vi "stageTriggerCam.vi"() -> ()   [LabVIEW 2015]
panel:
  in  "initTrigPos (mm)":dbl
  out "Frame Count":i32=1
  in  "File":path=path "C:/Users/sims01/Desktop/triggering1711/imgStack"
  in  "System no.":i32=2 min=1 step=1
  in  "zIdx":i32=1
  in  "error in":errorcluster
  in  "triggOutputIdx":string="3"
  in  "initPos (mm)":dbl
  in  "finPos (mm)":dbl=10.0
  in  "stepSize (mm)":dbl=0.5
  in  "motionSelection":enum32{"stop/ start", "cont."}(radio)=enum."cont."
  out "error out":errorcluster
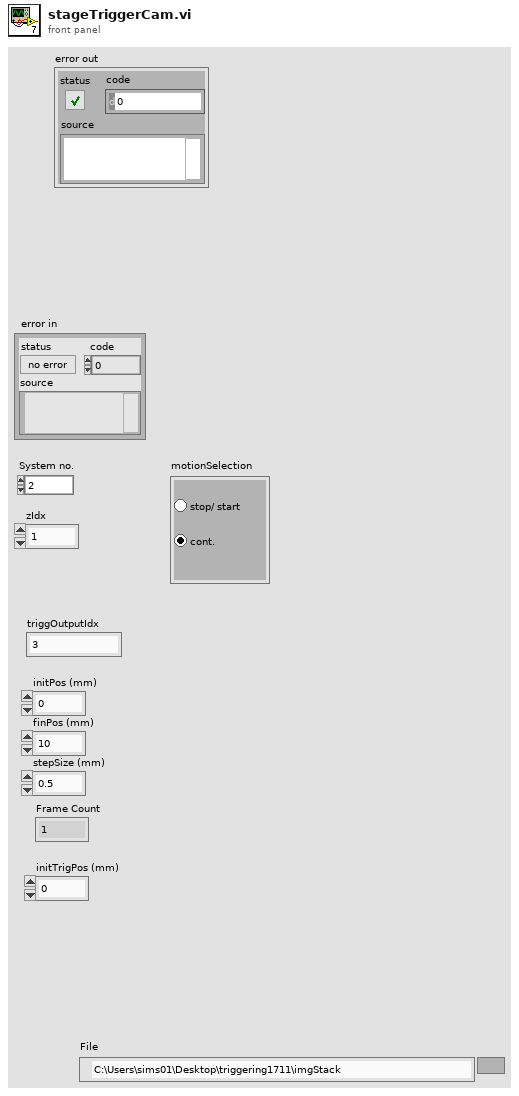
[diagram p1: front panel]
types:
  T1 = cluster{"Mode":u32, "Polarity":u32, "Times":u32, "Delay":dbl}
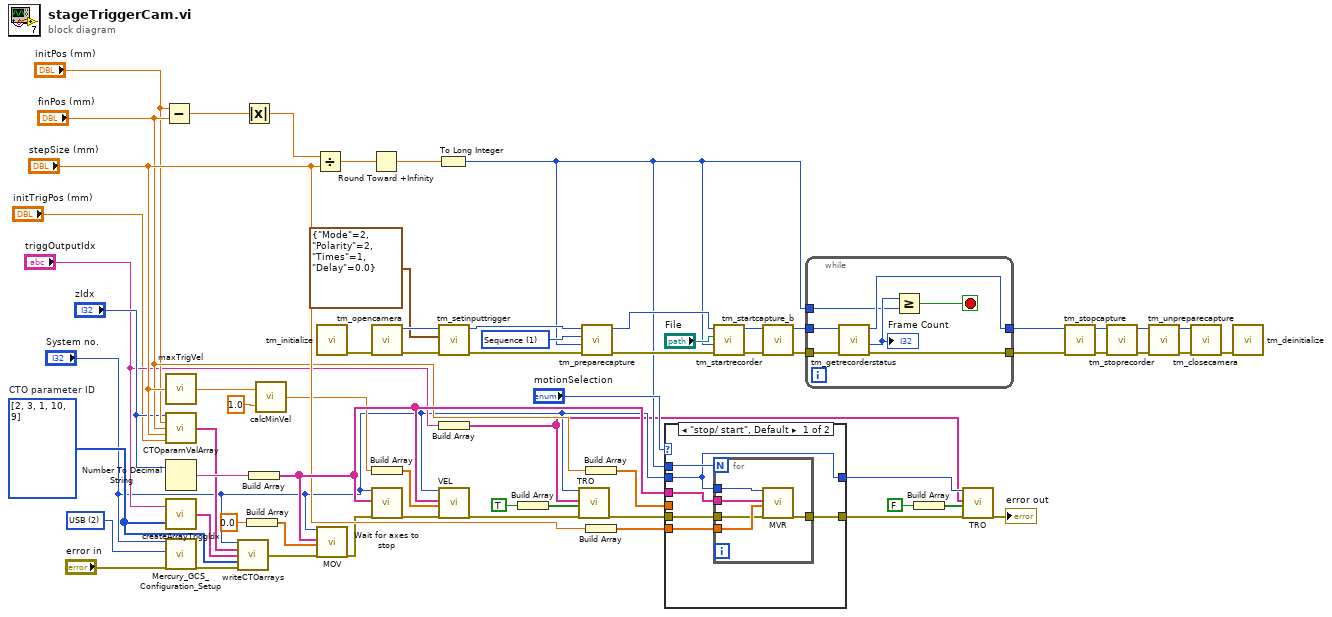
[diagram p0: block diagram]
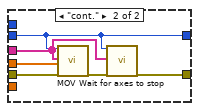
[diagram p2: hidden frame]
diagram:
  w35 = 1 items=["Snap", "Sequence"] ("Capture mode")
  w43 = i32[] [2, 3, 1, 10, 9]  # CTO parameter ID
  w41 = u16 2 items=["RS232", "RS232 DaisyChain", "USB", "USB_DaisyChain"] ("Interface")
  n1 = Subtract(x="initPos (mm)", y="finPos (mm)") -> (x-y=w60:dbl)
  n2 = call "maxTrigVel.vi"("stepSize (mm)"="stepSize (mm)") -> ("maxVel (mm/s)"=w50:dbl)
  n3 = call "CTOparamValArray.vi"("zIdx"="zIdx", "initPos (mm)"="initPos (mm)", "finPos (mm)"="finPos (mm)", "stepSize (mm)"="stepSize (mm)", "initTrigPos (mm)"="initTrigPos (mm)") -> ("CTOparamValArray"=w44:string[])  [unwired: 10 in]
  n4 = Number To Decimal String(number="zIdx") -> (decimal integer string=w49:string)  [unwired: 1 in]
  n5 = call "createArrayTriggIdx.vi"("CTO parameter ID"=w43, "triggOutputIdx"="triggOutputIdx") -> ("Array"=w42:string[])
  n6 = call "Mercury_GCS_Configuration_Setup.vi"("System no."="System no.", "Interface"=w41, "error in"="error in") -> ("error out"=w45:errorcluster)  [unwired: 10 in, 6 out]
  n7 = call "writeCTOarrays.vi"("System no."="System no.", "CTOparamValArray"=w44, "triggIdxArray"=w42, "CTO parameter ID"=w43, "error in"=w45) -> ("error out"=w16:errorcluster)  [unwired: 10 in]
  n8 = Absolute Value(x=w60) -> (abs(x)=w61:dbl)
  n9 = Build Array(0.0 ("element")) -> (w1:dbl[])
  n10 = Build Array(w49) -> (w65:string[])
  n11 = call "calcMinVel.vi"("velocity2"=1.0, "velocity1"=w50) -> ("minVal"=w52:dbl)
  n12 = Divide(x=w61, y="stepSize (mm)") -> (x/y=w62:dbl)
  n13 = call <userlib>:"tm_initialize.vi"() -> ("error out"=w39:errorcluster)  [unwired: 8 in, 3 out]
  n14 = call "MOV.vi"("System no."="System no.", "Axes to move"=w65, "Position values"=w1, "error in"=w16) -> ("error out"=w47:errorcluster)  [unwired: 15 in]
  n15 = Round Toward +Infinity(x=w62) -> (ceil(x): smallest int >= x=w57:dbl)
  n16 = call <userlib>:"tm_opencamera.vi"("error in (no error)"=w39) -> ("error out"=w30:errorcluster, "Handle out"=w38:u32)  [unwired: 8 in, 1 out]
  n17 = Build Array(w52) -> (w53:dbl[])
  n18 = call "Wait for axes to stop.vi"("System no."="System no.", "Axes to wait for"=w65, "error in"=w47) -> ("error out"=w54:errorcluster)  [unwired: 4 in, 12 out]
  n19 = To Long Integer(number=w57) -> (32bit integer=w13:i32)
  n20 = call <userlib>:"tm_setinputtrigger.vi"("error in (no error)"=w30, "Parameters"=T1 {"Mode"=2, "Polarity"=2, "Times"=1, "Delay"=0.0}, "Handle in"=w38) -> ("error out"=w29:errorcluster, "Handle out"=w36:u32)  [unwired: 7 in]
  n21 = Build Array("triggOutputIdx") -> (w8:string[])
  n22 = call "VEL.vi"("System no."="System no.", "Axes to set"=w65, "Velocity values"=w53, "error in"=w54) -> ("error out"=w14:errorcluster)  [unwired: 14 in, 1 out]
  n23 = Build Array(TRUE) -> (w7:bool[])
  n24 = call "TRO.vi"("System no."="System no.", "TriggerOut to command"=w8, "Trigger status"=w7, "error in"=w14) -> ("error out"=w15:errorcluster)  [unwired: 15 in]
  n25 = call <userlib>:"tm_preparecapture.vi"("error in (no error)"=w29, "Frames"=w13, "Capture mode"=w35, "Handle in"=w36) -> ("error out"=w24:errorcluster, "Handle out"=w25:u32)  [unwired: 4 in, 2 out]
  n26 = Build Array("finPos (mm)") -> (w56:dbl[])
  n27 = Build Array("stepSize (mm)") -> (w64:dbl[])
  n28 = case shown="\"stop/ start\", Default" "motionSelection" {
    tunnel: "System no." -> [w66 w77]
    tunnel: w65 -> [w70 w79]
    tunnel: w56 -> [_ w82]
    tunnel: w15 -> [w68 w81]
    tunnel: [w67 w78] -> w11
    tunnel: w13 -> [w71 _]
    tunnel: w64 -> [w69 _]
    tunnel: [w66 w77] -> w9
    frame "stop/ start", Default {
      n29 = for {
        N: w71 -> [_]
        tunnel: w66 -> [w76]
        tunnel: w70 -> [w75]
        tunnel: w69 -> [w74]
        tunnel: w68 -> [w73]
        tunnel: [w72] -> w67
        n30 = call "MVR.vi"("System no."=w76, "Axes to move"=w75, "Position values"=w74, "error in"=w73) -> ("error out"=w72:errorcluster)  [unwired: 1 in, 14 out]
      }
    }
    frame "cont." {
      n31 = call "MOV.vi"("System no."=w77, "Axes to move"=w79, "Position values"=w82, "error in"=w81) -> ("error out"=w80:errorcluster)  [unwired: 15 in]
      n32 = call "Wait for axes to stop.vi"("System no."=w77, "Axes to wait for"=w79, "error in"=w80) -> ("error out"=w78:errorcluster)  [unwired: 4 in, 12 out]
    }
  }
  n33 = call <userlib>:"tm_startrecorder.vi"("error in (no error)"=w24, "frames"=w13, "File"="File", "Handle in"=w25) -> ("error out"=w26:errorcluster, "Handle out"=w27:u32)  [unwired: 6 in]
  n34 = call <userlib>:"tm_startcapture_b.vi"("error in (no error)"=w26, "Handle in"=w27) -> ("error out"=w22:errorcluster, "Handle out"=w23:u32)  [unwired: 8 in]
  n35 = while {
    tunnel: w13 -> [w84]
    tunnel: [w87] -> w32
    tunnel: [w86] -> w28
    tunnel: w23 -> [w89]
    tunnel: w22 -> [w88]
    stop <- w83 stop-if-true
    n36 = call <userlib>:"tm_getrecorderstatus.vi"("error in (no error)"=w88, "Handle"=w89) -> ("error out"=w86:errorcluster, "Count"=w85:i32, "Handle"=w87:u32)  [unwired: 6 in, 1 out]
    "Frame Count" <- w85
    n37 = Greater Or Equal?(x=w85, y=w84) -> (x >= y?=w83:bool)
  }
  n38 = Build Array(FALSE) -> (w4:bool[])
  n39 = call "TRO.vi"("System no."=w9, "TriggerOut to command"=w8, "Trigger status"=w4, "error in"=w11) -> ("error out"=→"error out":errorcluster)  [unwired: 15 in]
  n40 = call <userlib>:"tm_stopcapture.vi"("error in (no error)"=w28, "Handle in"=w32) -> ("error out"=w20:errorcluster, "Handle out"=w21:u32)  [unwired: 8 in]
  n41 = call <userlib>:"tm_stoprecorder.vi"("error in (no error)"=w20, "Handle in"=w21) -> ("error out"=w18:errorcluster, "Handle out"=w19:u32)  [unwired: 8 in]
  n42 = call <userlib>:"tm_unpreparecapture.vi"("error in (no error)"=w18, "Handle in"=w19) -> ("error out"=w33:errorcluster, "Handle out"=w31:u32)  [unwired: 8 in]
  n43 = call <userlib>:"tm_closecamera.vi"("error in (no error)"=w33, "Handle in"=w31) -> ("error out"=w34:errorcluster)  [unwired: 9 in]
  n44 = call <userlib>:"tm_deinitialize.vi"("error in (no error)"=w34) -> ()  [unwired: 10 in, 1 out]
